vi "Log If Error.vi"(4 "Include Warnings(F)":bool, 6 "Clear After Logging?(F)":bool, 7 "Event Level (Error)":T1=enum."Error", 8 "error in (no error)":errorcluster, 10 "SourceID":string, 11 "Logger in":refnum<class "Logger.lvclass">) -> (0 "error out":errorcluster, 3 "Logger out":refnum<class "Logger.lvclass">)   [LabVIEW 2020, in "Event Log.lvlib" / "Logger.lvclass"]
uses:
  Logger.lvclass
  <vilib>/gpm_packages/@cs/event-logger/Source/Composed Log/Types/Log Level.ctl
  Logger.lvclass/Logger.ctl
  <vilib>/gpm_packages/@cs/event-logger/Source/Composed Log/LoggerReference/LoggerReference.lvclass
  <vilib>/gpm_packages/@cs/event-logger/Source/Composed Log/Composed Log.lvlib
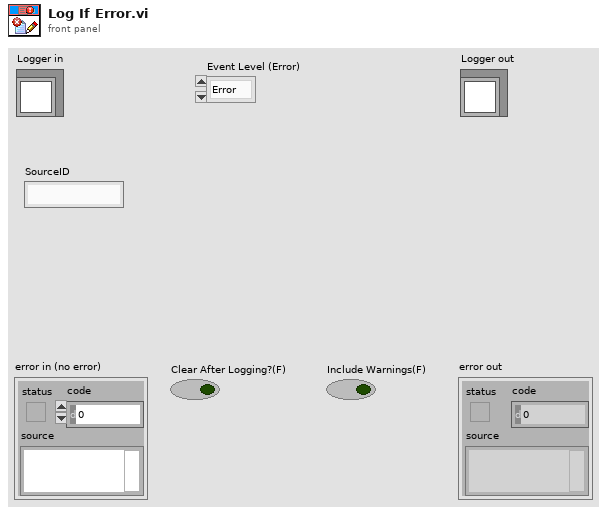
[diagram p1: front panel]
types:
  T1 = typedef "Composed Log.lvlib/Log Level.ctl" = enum16{"Debug", "Info", "Warning", "Error", "Critical"}
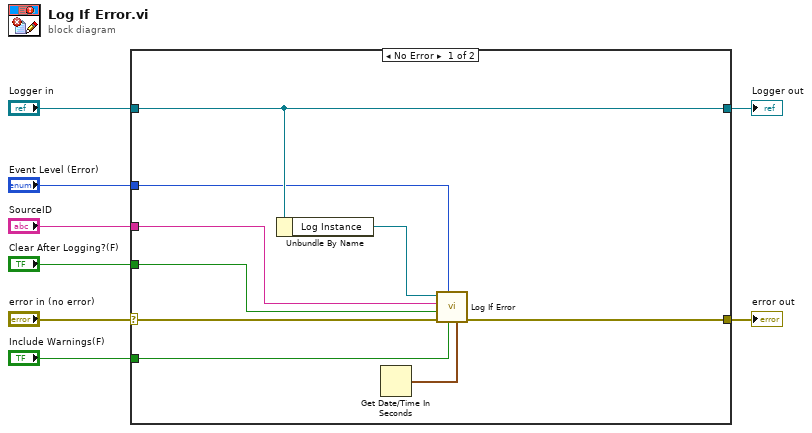
[diagram p0: block diagram]
diagram:
  n1 = case shown="No Error" "error in (no error)" {
    selector: "error in (no error)" -> [w15 w19]
    tunnel: [w14 w19] -> w7
    tunnel: [w17 w18] -> w5
    tunnel: "Logger in" -> [w17 w18]
    tunnel: "Include Warnings(F)" -> [w13 _]
    tunnel: "Event Level (Error)" -> [w12 _]
    tunnel: "SourceID" -> [w11 _]
    tunnel: "Clear After Logging?(F)" -> [w10 _]
    frame No Error {
      n2 = Unbundle By Name(w17) -> ("Log Instance"=w16:refnum<class "LoggerReference.lvclass">)
      n3 = Get Date/Time In Seconds() -> (seconds since 1Jan1904=w9:timestamp)
      n4 = call <vilib>:"Log If Error.vi"("Event Time"=w9, "Include Warnings(F)"=w13, "Event Level (Error)"=w12, "Error In"=w15, "Clear After Logging?(F)"=w10, "SourceID"=w11, "Log Instance"=w16) -> ("error out"=w14:errorcluster)  [unwired: 3 in, 1 out]
    }
    frame Error {
    }
  }
  "error out" <- w7
  "Logger out" <- w5
